vi "ValidateUser.vi"(4 "error in (no error)":errorcluster, 5 "password":string, 6 "username":string, 7 "configuration file path":path) -> (0 "error out":errorcluster, 1 "Valid Password?":bool, 2 "User Type":T1, 3 "configuration file path dup":path)   [LabVIEW 2015]
uses:
  GUI/GUI_states.ctl
  <vilib>/Utility/config.llb/Read Key (String).vi
  <vilib>/Utility/config.llb/Read Key (I32).vi
  <vilib>/Utility/config.llb/NI_LVConfig.lvlib
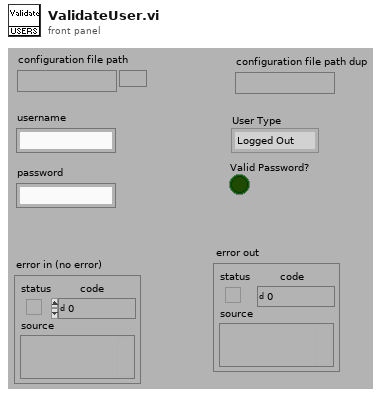
[diagram p1: front panel]
types:
  T1 = typedef "GUI_states.ctl" = enum16{"Logged Out", "Observer", "Operator", "Engineer"}
  T2 = typedef "NI_LVConfig.lvlib/Config Data RefNum.ctl" = refnum<k1>
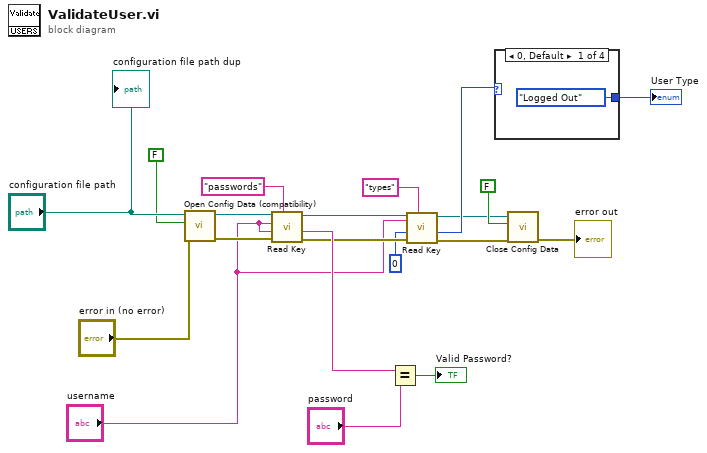
[diagram p0: block diagram]
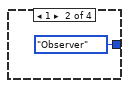
[diagram p2: hidden frame]
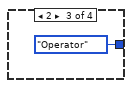
[diagram p3: hidden frame]
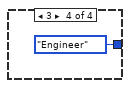
[diagram p4: hidden frame]
diagram:
  n1 = call <vilib>:"Open Config Data (compatibility).vi"("error in (no error)"="error in (no error)", "create file if necessary (T)"=FALSE, "configuration file path"="configuration file path") -> ("error out"=w16:errorcluster, "refnum"=w17:T2)  [unwired: 6 in, 1 out]
  n2 = call-poly <vilib>:"Read Key.vi"("section"="passwords", "error in (no error)"=w16, "default value"="username", "key"="username", "refnum"=w17) -> ("error out"=w10:errorcluster, "value"=w12:string, "refnum out"=w9:T2)  [unwired: 3 in, 1 out]
  n3 = Equal?(x=w12, y="password") -> (x = y?=→"Valid Password?":bool)
  n4 = call-poly <vilib>:"Read Key.vi"("section"="types", "error in (no error)"=w10, "default value"=0, "key"="username", "refnum"=w9) -> ("error out"=w2:errorcluster, "value"=w5:i32, "refnum out"=w3:T2)  [unwired: 3 in, 1 out]
  n5 = case shown="0, Default" w5 {
    tunnel: [GUI_states."Logged Out" ("User Type") GUI_states."Observer" ("User Type") GUI_states."Operator" ("User Type") GUI_states."Engineer" ("User Type")] -> w4
    frame 0, Default {
    }
    frame 1 {
    }
    frame 2 {
    }
    frame 3 {
    }
  }
  "User Type" <- w4
  n6 = call <vilib>:"Close Config Data.vi"("error in (no error)"=w2, "write file if changed (T)"=FALSE, "refnum"=w3) -> ("error out"=→"error out":errorcluster)  [unwired: 7 in, 1 out]
  "configuration file path dup" <- "configuration file path"
